vi "simx Get Dialog Input.vi"(7 "operationMode":i32, 8 "error in (no error)":errorcluster, 9 "inputText":string, 10 "dialogHandle":i32, 11 "clientID":i32) -> (0 "error out":errorcluster, 1 "inputText out":string, 3 "function return":i32)   [LabVIEW 2019, in "PXL_V-REP.lvlib"]
doc: "EXTAPI_DLLEXPORT simxInt simxGetDialogInput(simxInt clientID,simxInt dialogHandle,simxChar** inputText,simxInt operationMode);"
uses:
  PXL_V-REP.lvlib
  <userlib>/V-REP/remoteApi.dll
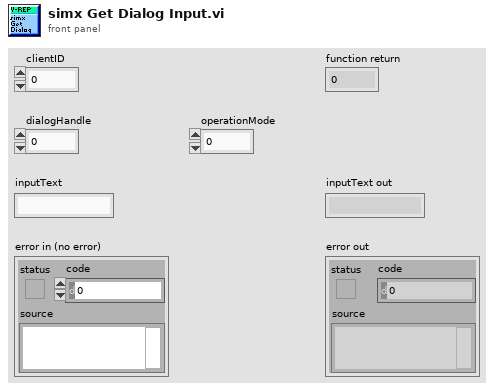
[diagram p1: front panel]
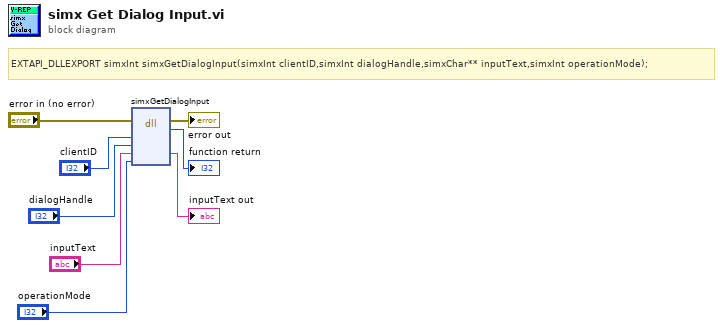
[diagram p0: block diagram]
diagram:
  # "EXTAPI_DLLEXPORT simxInt simxGetDialogInput(simxInt clientID,simxInt dialogHandle,simxChar** inputText,simxInt operationMode);"
  n1 = dll-call lib="C:/Program Files (x86)/National Instruments/LabVIEW 2019/user.lib/V-REP/remoteApi.*" fn="simxGetDialogInput"(error in="error in (no error)", "clientID"="clientID", "dialogHandle"="dialogHandle", "inputText"="inputText", "operationMode"="operationMode") -> (error out=→"error out":errorcluster, →"function return":i32, "inputText"=→"inputText out":string)  [unwired: 5 in, 1 out]
